vi "Device2.vi"() -> ()   [LabVIEW 2017]
uses:
  D:/upwork/Laser Measurement Tool/Laser/tests/KIM101/Thorlabs.MotionControl.Controls.dll
  Thorlabs.MotionControl.Controls.dll
panel:
  out "CreateDevice":bool
  in  "ChannelNumber":i32=1
  out "error out":errorcluster
  in  "stop":bool
  in  "SerialNumber":string="97000001"
  # "Without UI test"
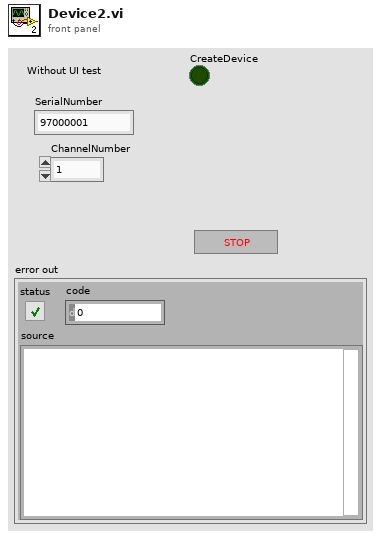
[diagram p1: front panel]
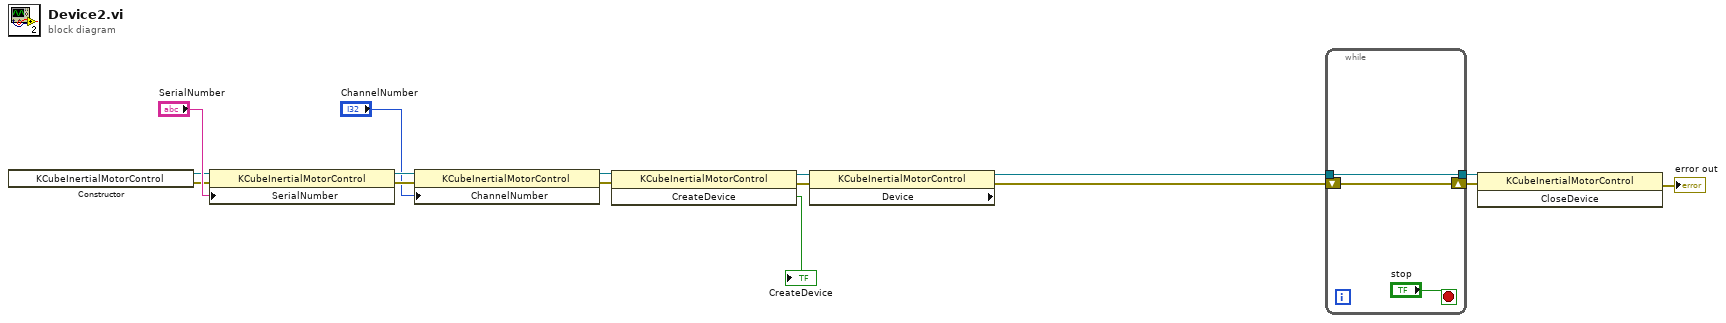
[diagram p0: block diagram]
diagram:
  n1 = constructor class="KCubeInertialMotorControl"() -> (reference out=w15:refnum<k24>, error out=w14:errorcluster)  [unwired: 3 in, 1 out]
  n2 = property class="KCubeInertialMotorControl"(reference=w15, error in=w14, "SerialNumber"="SerialNumber") -> (reference out=w9:refnum<k24>, error out=w10:errorcluster)
  n3 = property class="KCubeInertialMotorControl"(reference=w9, error in=w10, "ChannelNumber"="ChannelNumber") -> (reference out=w6:refnum<k24>, error out=w7:errorcluster)
  n4 = invoke class="KCubeInertialMotorControl" method="CreateDevice"(reference=w6, error in=w7) -> (reference out=w4:refnum<k24>, error out=w5:errorcluster, "CreateDevice"=→"CreateDevice":bool)  [unwired: 1 in]
  n5 = property class="KCubeInertialMotorControl" props=["Device"](reference=w4, error in=w5) -> (reference out=w3:refnum<k24>, error out=w2:errorcluster)  [unwired: 1 out]
  n6 = while {
    tunnel: w3 -> [w18]
    shift-right: [w19] -> w13
    shift-left: w2 -> [w19]
    tunnel: [w18] -> w12
    stop <- "stop" stop-if-true
  }
  n7 = invoke class="KCubeInertialMotorControl" method="CloseDevice"(reference=w12, error in=w13) -> (error out=→"error out":errorcluster)  [unwired: 1 in, 2 out]
